vi "AlliGator Draw Phasor Ratio References on Phasor Plot.vi"(8 "error in (no error)":errorcluster, 9 "Overlay Group":string="Phasor Ratio References", 11 "Phasor Plot Refnum in":T1) -> (0 "error out":errorcluster, 3 "Phasor Plot Refnum out":T1)   [LabVIEW 2021, in "AlliGator Phasor Plot.lvlib"]
doc: "Does the actual drawing of Phasor Ratio References (and associated segment and boundary region) on the Phasor Plot image."
uses:
  AlliGator Phasor Plot.lvlib
  <vilib>/vision/Image Controls.llb/IMAQ Image.ctl
  Globals, Variables, Constants/AlliGator Variables List.ctl
  Phasor Ratio/AlliGator Phasor Plot Reference Points.ctl
  Settings/AlliGator Settings List.ctl
  08c29e31-a428-4f06-8fa9-37cc1cf687de.vi
  a2f43300-ec38-48b4-b16a-acb1cf69b6dd.vi
  Variant/Variant to Data/Variant to DBL.vi
  Variant/Variant to Data/Variant to I32.vi
  Variant/Variant to Data/Variant to Boolean.vi
  Globals, Variables, Constants/AlliGator Globals, Variables & Constants.lvlib
  Phasor Ratio/AlliGator Phasor Ratio.lvlib
  Settings/AlliGator Settings.lvlib
  Variant/Variant to Data/Variant to Data.lvlib
  Time/Time.lvlib
  Image/Image.lvlib
  Error/Error.lvlib
panel:
  out "elapsed (relative) seconds":dbl
  # "see the AlliGator License on the block diagram (Ctrl+E or Window:Show Block Diagram)"
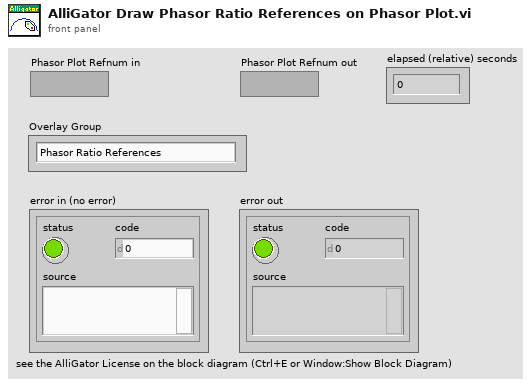
[diagram p1: front panel]
types:
  T1 = typedef "IMAQ Image.ctl" = refnum<image>
  T2 = typedef "IMAQ Point" = cluster{"X":sgl, "Y":sgl}
  T3 = typedef "AlliGator Settings.lvlib/AlliGator Settings List.ctl" = enum16{"GUI:Visible Settings Tab", "GUI:Last Run Version", "Source Image:Use Image Histogram for Contrast", "Source Image:Low Count Pixels Rejection Options", "Source Image:High Count Pixels Rejection Options", "Source Image:Use Image Brightness", "Source Image:Blend Overlay with Image Background", "Source Image:Use Fixed ROI Diameter", "Source Image:ROI Diameter", "Source Image:ROI Center Color", "Source Image:Peak Threshold", "Source Image:Intensity Threshold", "Source Image:Image Binning Options", "Source Image:Image Smoothing Options", "Source Image:Image Histogram Active", "Source Image:Invert Binary Mask", "Source Image:Hot Pixel Removal", "Source Image:Overlay Analyzed ROI Center", "Source Image:Auto-Adjust Contrast", "Source Image:Histogram Lower Percentile", "Source Image:Histogram Upper Percentile", "Source Image:Save Source Image", "Source Image:Scale Bar Options", "Source Image:Image Resolution (Pixel Size)", "Source Image:Flatfield Correction", "Source Image:Show Dead Left Columns Correction", "Source Image:Dead Left Columns Correction", "Source Image:Image Pre-Processing Operations Order", "Source Image:Overlay ROI Median", "Source Image:Median Overlay Color", "Data Information:Gate Width", "Data Information:Nanotime Gate Separation", "Data Information:Macrotime Gate Separation", "Data Information:Gate Step", "Data Information:# Gates", "Data Information:Gate Image Exposure", "Data Information:Gate Image Integration", "Data Information:Gates to Skip", "Data Information:Gates to Keep", "Data Information:Define Gates to", "Data Information:Channel Name", "Data Information:Available Channel Names", "Data Information:Channel Arithmetic", "Data Information:Background File Subtraction", "Data Information:Background File", "Data Information:Background Scaling Factor", "Data Information:Background Pile-up Correction", "Data Information:Background Pixel Well Capacity", "Data Information:Laser Period", "Data Information:SYNC Period", "Data Information:Pile-up Correction", "Data Information:Pixel Well Capacity", "Data Information:Dataset Scaling Factor", "Fluorescence Decay_Decay Pre-Processing:Reverse Gates", "Fluorescence Decay_Decay Pre-Processing:Verbose Decay Pre-Processing", "Fluorescence Decay_Decay Pre-Processing:Use Decay Pre-Processing", "Fluorescence Decay_Decay Pre-Processing:Background Subtraction", "Fluorescence Decay_Decay Pre-Processing:Background Definition Range", "Fluorescence Decay_Decay Pre-Processing:Baseline Subtraction Method", "Fluorescence Decay_Decay Pre-Processing:Decay Pre-Processing Operations Order", "Fluorescence Decay_Decay Pre-Processing:Smoothing Parameter", "Fluorescence Decay_Decay Pre-Processing:Shift Decay", "Fluorescence Decay_Decay Pre-Processing:Decay Shift Parameters", "Fluorescence Decay_Decay Pre-Processing:Fold Decay", "Fluorescence Decay_Decay Pre-Processing:# Folds", "Fluorescence Decay_Decay Pre-Processing:1-Normalize Decay", "Fluorescence Decay_Decay Pre-Processing:[0-1]-Normalize Decay", "Fluorescence Decay_Decay Pre-Processing:Smoothen Decay", "Fluorescence Decay_Decay Pre-Processing:Extrapolate Decay", "Fluorescence Decay_Decay Pre-Processing:Use Periodicity", "Fluorescence Decay_Decay Pre-Processing:Use Cursors", "Fluorescence Decay_Decay Pre-Processing:Tail Fraction", "Fluorescence Decay_Decay Pre-Processing:Head Fraction", "Fluorescence Decay_Decay Pre-Processing:Additional Points", "Fluorescence Decay_Decay Pre-Processing:Straighten Decay", "Fluorescence Decay_Decay Pre-Processing:Constant Background", "Fluorescence Decay_Decay Pre-Processing:Pixel-Normalize Decay", "Fluorescence Decay_Advanced Analysis:Extract IRF instead of Decay", "Fluorescence Decay_Advanced Analysis:IRF Extraction Options", "Fluorescence Decay_Advanced Analysis:IRF Optimization Options", "Fluorescence Decay_Advanced Analysis:Square Pulse Options", "Fluorescence Decay_Advanced Analysis:IRF Order", "Fluorescence Decay_Advanced Analysis:IRF Time Constants", "Fluorescence Decay_Advanced Analysis:Wavelet Analysis Options", "Fluorescence Decay_Advanced Analysis:Average Lifetime Options", "Fluorescence Decay_Fit Options:Fit Options", "Fluorescence Decay_Fit Options:Use Legacy Fitting Approach", "Fluorescence Decay_Fit Options:Use Data Information Laser Period", "Fluorescence Decay_Fit Parameters:Displayed Fit Parameters", "Fluorescence Decay_Fit Parameters:Fit Parameter Constraints", "Fluorescence Decay_Fit Parameters:Export Tabulated Results", "Fluorescence Decay_Fit Parameters:MLE Baseline Offset Type", "Fluorescence Decay_Fit Parameters:MLE Baseline Offset", "Fluorescence Decay_Fit Parameters:Guess Parameter Names", "Fluorescence Decay_Fit Parameters:Guess Parameter Values", "Fluorescence Decay_Fit Parameters:Guess Parameters Options", "Fluorescence Decay_Fit Parameters:Optimal Offset Selection Criterion", "Fluorescence Decay_Styles:Show Last Decay Only", "Fluorescence Decay_Styles:Decay Graph Color Array", "Fluorescence Decay:Decay Graph Active", "Fluorescence Decay Statistics:Min Peak Value", "Fluorescence Decay Statistics:Reject Low Decay Peak Pixels", "Fluorescence Decay Statistics:Reject High Decay Peak Pixels", "Fluorescence Decay Statistics:Max Peak Value", "Time Traces:Use File Timestamp", "Time Traces:Time Step", "Time Traces:Use Intensity Correction File", "Time Traces:Intensity Correction File", "Phasor Plot:Phasor Plot Smoothing Options", "Phasor Plot:Phasor Plot Size", "Phasor Plot:Phasor Plot Graphics Options", "Phasor Plot:Cumulative Phasor Plot", "Phasor Plot:Use Phasor Brightness", "Phasor Plot:Blend Overlay with Phasor Background", "Phasor Plot:Save Phasor Plot", "Phasor Plot:Show References", "Phasor Plot:Phasor Ratio Decay Range", "Phasor Plot:Exponential Fading", "Phasor Plot:Phasor Ratio Reference Colors", "Phasor Plot:Reference Radius", "Phasor Plot:Show Color Map Vertices", "Phasor Plot:Phasor Plot Active", "Phasor Plot:Phasor Ratio Color Map Type", "Phasor Plot:Phasor Ratio Color Map", "Phasor Plot:Phasor Ratio Display Range", "Phasor Plot:Selected Image ROI(s)", "Phasor Plot:All Image ROIs", "Phasor Plot:Selected Phasor Plot ROI(s)", "Phasor Plot:All Phasor Plot ROIs", "Phasor Plot:Phasor Ratio Color-Coded Quantity", "Phasor Plot:Store Phasor Harmonics", "Phasor Plot:Draw Reference Segment", "Phasor Plot:User-Defined Quantity", "Phasor Plot:Color Scale High Color", "Phasor Plot:Color Scale Low Color", "Phasor Plot:Intensity-weighted Phasor Plot", "Phasor Graph:Phasor Frequency", "Phasor Graph:Phasor Ratio Type", "Phasor Graph:Pixel-level Phasor Computation", "Phasor Graph:Save Phasor Graph", "Phasor Graph:Phasor Graph Active", "Phasor Graph:Phasor SDV Options", "Phasor Graph:Intensity-weighted Phasor Graph", "Phasor Graph:Define Shortest Lifetime as", "Phasor Calibration:Use Backup Calibration if needed", "Phasor Calibration:Backup Calibration Type", "Phasor Calibration:Calibration Type", "Phasor Calibration:Calibration Lifetime", "Phasor Calibration:Calibration Map Algorithm", "Single-Exponential Phasor Locus (SEPL):Gate Parameters", "Single-Exponential Phasor Locus (SEPL):User-defined Gate", "Single-Exponential Phasor Locus (SEPL):User-defined IRF", "Single-Exponential Phasor Locus (SEPL):Phasor Parameters", "Single-Exponential Phasor Locus (SEPL):Decay & IRF Parameters", "Single-Exponential Phasor Locus (SEPL):Display Parameters", "Lifetime Analysis:Decay Analysis Parameters", "Lifetime Analysis:Lifetime Map Active", "Plugins:Python Settings", "Miscellaneous:Verbose Mode", "Miscellaneous:Beep after Script", "Miscellaneous:Saved Image File Format", "Miscellaneous:Exported Gate Image Settings", "Miscellaneous:Include Loading in Timing", "Miscellaneous:Verbose Settings Mode", "Miscellaneous:Histogram Options", "Miscellaneous:Beep on Error", "Miscellaneous:# Logical Processors Used", "Miscellaneous:ROI Description Max Characters", "Miscellaneous:Verbose Error Mode", "Miscellaneous:Transparent Mask Color"}
  T4 = cluster{"Reference 1":u32, "Reference 2":u32, "Boundary":u32}
  T5 = typedef "AlliGator Phasor Ratio.lvlib/AlliGator Phasor Plot Reference Points.ctl" = cluster{"O_h":dbl, "O_v":dbl, "1_h":dbl, "1_v":dbl}
  T6 = typedef "AlliGator Globals, Variables & Constants.lvlib/AlliGator Variables List.ctl" = enum16{"---- GUI ----", "GUI:Initialization Status", "GUI:State Indicators Refnum", "GUI:Original AlliGator Menu Items", "GUI:Current Action Loop State", "GUI:Script in progress", "GUI:Playback", "GUI:Loop Playback", "GUI:Search ROI Used", "GUI:Search ROI", "Decay Graph Max Legend Size", "Intensity Graph Max Legend Size", "Decay Statistics Graph Max Legend Size", "Phasor Graph Max Legend Size", "Phasor Ratio Graph Max Legend Size", "Lifetime Graph Max Legend Size", "---- Files ----", "Files:Export Dataset Frames as Individual Files", "Files:Show Batch Export Help Balloons", "Files:Frames in Dataset", "Files:ptu File Frame Start Indices", "Files:Current Frame in Dataset", "Files:Current Frame Timestamp", "Files:Dataset Loaded", "Files:Dataset Metadata", "Files:Dataset Channel", "Files:Dataset Data Description", "Files:Background Dataset Metadata", "Files:Background Dataset Channel", "Files:Background Dataset Data Description", "Files:Background File Subtraction", "Files:Background File Path", "Files:Background File Pile-up Correction", "Files:Background File Pixel Well Capacity", "Files:Background File Scaling Factor", "Files:Current Dataset Load Settings", "Files:Dataset Path", "Files:ICCD-specific Information", "Files:Macrotime Gate Separation", "------ Python Plugins ------", "Python Plugins:Information", "Python Plugins:Python Session", "Python Plugins:Valid Python Session?", "---- Source Image ----", "Source Image:ROIs", "Source Image:Current ROI", "Source Image:ROI Event Refnum", "X_Source Image:Display Range", "X_Source Image:Palette Information", "X_Source Image:Type of Displayed Image", "X_Time Gate Slider", "Source Image:Palette List", "Source Image:Scale", "Source Image:ROI Overlay Color", "Source Image:Overlay to Erase", "Source Image:Is Displayed Image Accumulated", "Source Image:White Light Image Modified", "Source Image:Mask Image Modified", "---- Image Profile Window ----", "Image Profile:Window Event Refnum", "Image Profile:IntensityType", "Image Profile:Intensity Average Type", "Image Profile:Intensity-weighted SDV", "Image Profile:Box Profile Type", "Image Profile:Window Open", "Image Profile:Plotted Fit Parameter", "------ Phasor Graph -------", "Phasor Graph:Show Line", "---- Phasor Plot ---", "Phasor Plot:Parameters Changed", "Phasor Plot:FLI Dataset Modified since last Calculation", "Phasor Harmonics Data", "Selected Phasor Harmonics", "Phasor Harmonic Manager Event Refnum", "Phasor Plot:ROIs", "Phasor Plot:Current ROI", "Phasor Plot:ROI Event Refnum", "Phasor Plot:Image Reference Points", "Phasor Plot:Computed", "Phasor Plot:Palette Information", "Phasor Plot:Palette List", "Phasor Plot:Phasor Ratio Palette Information", "Phasor Plot:Phasor Ratio Palette List", "Phasor Plot:Image Scale", "Phasor Plot:Image Overlay to Erase", "Phasor Plot:Image Elements to Update", "Phasor Plot:Current Calculation Parameters", "Phasor Plot:Current Calibration Options", "Phasor Plot:Reset Cumulated Phasor Plot", "Phasor Plot:Reference 1", "Phasor Plot:Lifetime Reference 1", "Phasor Plot:Reference 1 Frequency", "Phasor Plot:Reference 2", "Phasor Plot:Lifetime Reference 2", "Phasor Plot:Reference 2 Frequency", "---- Decay Analysis ----", "Number of Selected Decays to Fit", "LS Fit Results", "LAR Fit Results", "BS Fit Results", "Last Decay Max - Min", "Best Fit Parameters", "Best Fit Parameter Names", "Actual Size X", "Actual Size Y", "Binning X", "Binning Y", "Actual # Gates", "Dataset Number", "Gates to...", "Gates Skipped", "Gates to keep", "Gate Step", "Gate Separation", "Reversed Gates", "Pile-up Correction", "Pixel Well Capacity", "Background Subtracted", "Background Subtraction Method", "Background Definition Range", "Background File (deprecated)", "Number of Dataset Accumulated", "Array of Accumulated Dataset Paths", "Do Averaged Datasets", "Destination File Path", "Process Plot Target", "Use 1/D as Phasor Frequency", "---- Decay Fit Parameter Map -----", "Decay Fit Parameter Map:Palette Information", "Decay Fit Parameter Map:Palette List", "Decay Fit Parameter Map:X Resolution", "Decay Fit Parameter Map:Y Resolution", "Decay Fit Parameter Map:Use Decay Fit Result Constraints", "Decay Fit Parameter Map:Decay Fit Result Constraints", "Decay Fit Parameter Map:Decay Fit Result Constraints Applied", "---- Parameter Map ----", "Parameter Map:Palette Information", "Parameter Map:Palette List", "------- Local Decay Window ---------", "Local Decay Graph Window:Event Refnum", "Local Decay Graph Window:Use normalized IRF for convolution", "----- Miscellaneous ----", "Misc:Skippable Dialog Windows Status"}
  T7 = typedef "Phasor.lvlib/Phasor (g, s).ctl" = cluster{"g":dbl, "s":dbl}
  T8 = cluster{"Phasor Plot x":dbl, "Phasor Plot y":dbl}
  T9 = cluster{"Left":i32, "Top":i32, "Right":i32, "Bottom":i32}
  T10 = cluster{"Phasor Plot x":dbl, "Phasor Plot y":dbl}[]
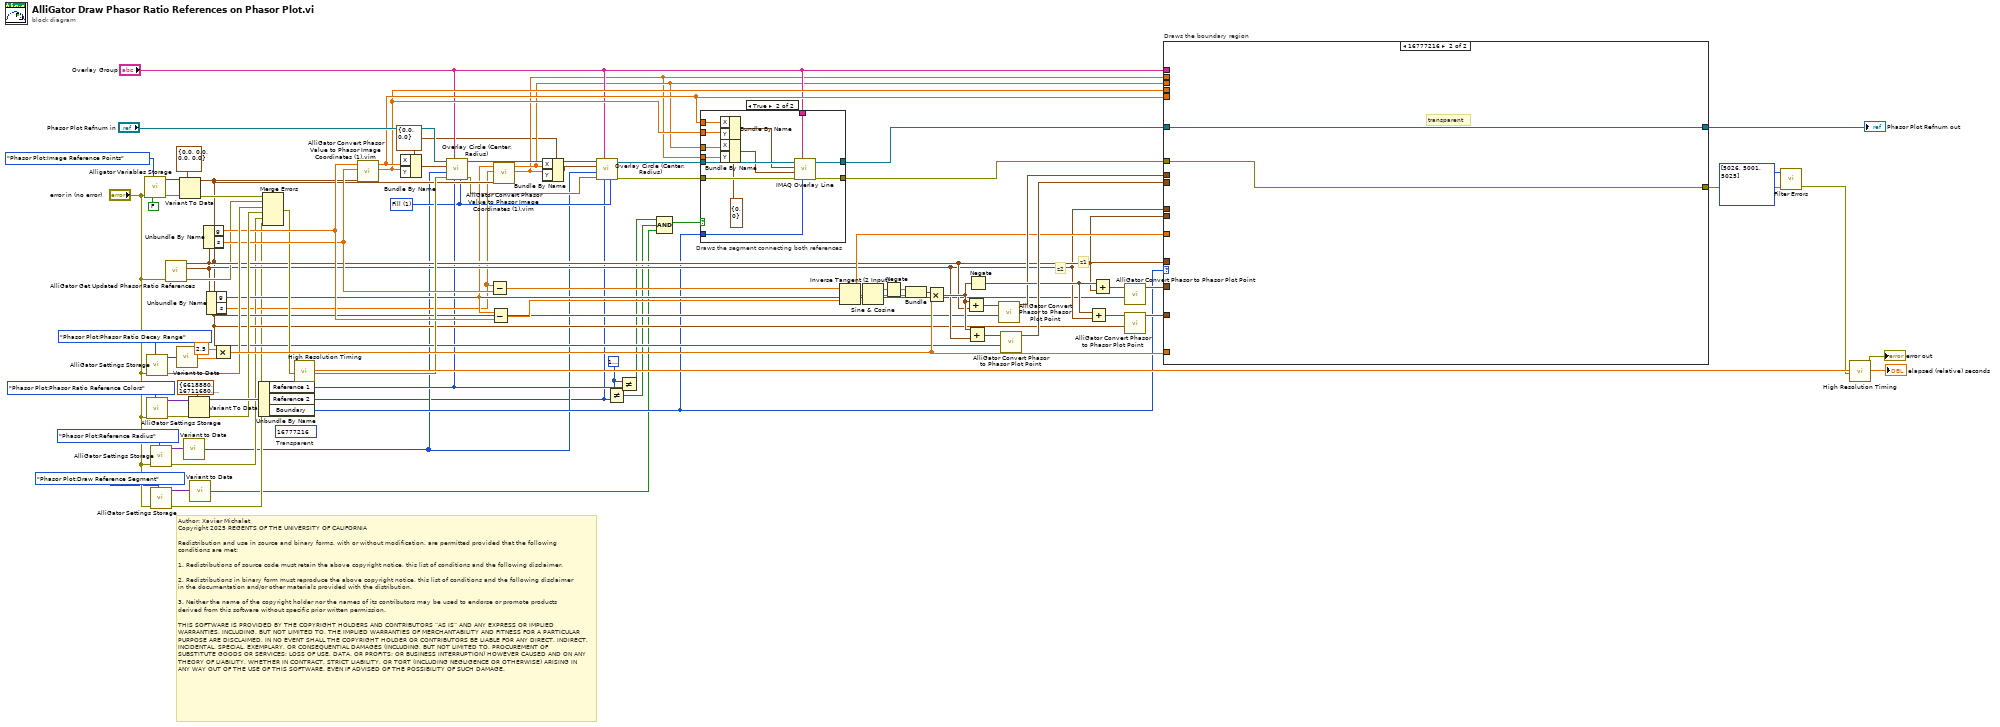
[diagram p0: block diagram]
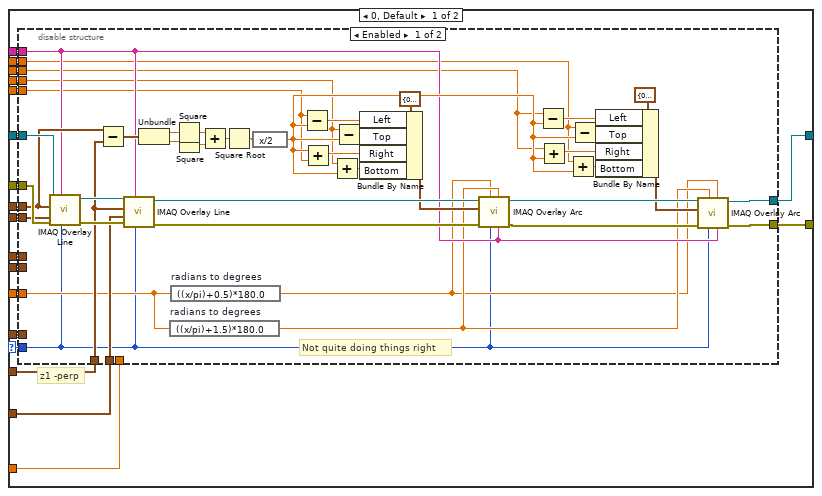
[diagram p3: hidden frame]
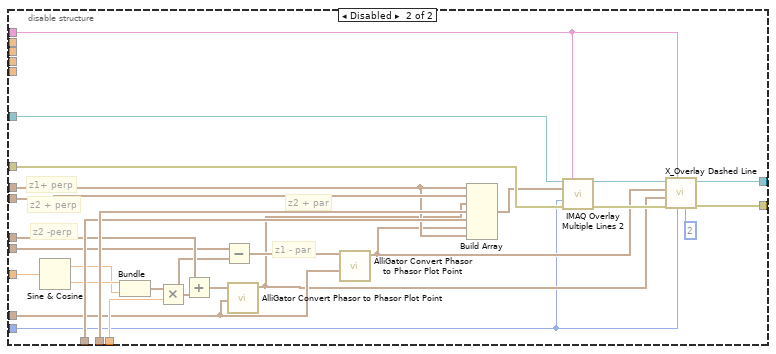
[diagram p4: hidden frame]
diagram:
  w3 = u32 1 items=["Frame", "Fill"] ("Drawing Mode (Frame)")
  w15 = u32 16777216 ("Color")
  w5 = T2 {"X"=0.0, "Y"=0.0} ("Center")
  (unwired) u32 16777216  # Transparent
  # "Author: Xavier Michalet\nCopyright 2025 REGENTS OF THE UNIVERSITY OF CALIFORNIA\n\nRedistribution and use in source and binary forms, with or without modification, are permitted provided that the following conditions are met:\n\n1. Redistributions of source code must retain the above copyright notice, this list of conditions and the following disclaimer.\n\n2. Redistributions in binary form must reproduce the above copyright notice, this list of conditions and the following disclaimer in the documentation and/or other materials provided with the distribution.\n\n3. Neither the name of the copyright holder nor the names of its contributors may be used to endorse or promote products derived from this software without specific prior written permission.\n\nTHIS SOFTWARE IS PROVIDED BY THE COPYRIGHT HOLDERS AND CONTRIBUTORS “AS IS” AND ANY EXPRESS OR IMPLIED WARRANTIES, INCLUDING, BUT NOT LIMITED TO, THE IMPLIED WARRANTIES OF MERCHANTABILITY AND FITNESS FOR A PARTICULAR PURPOSE ARE DISCLAIMED. IN NO EVENT SHALL THE COPYRIGHT HOLDER OR CONTRIBUTORS BE LIABLE FOR ANY DIRECT, INDIRECT, INCIDENTAL, SPECIAL, EXEMPLARY, OR CONSEQUENTIAL DAMAGES (INCLUDING, BUT NOT LIMITED TO, PROCUREMENT OF SUBSTITUTE GOODS OR SERVICES; LOSS OF USE, DATA, OR PROFITS; OR BUSINESS INTERRUPTION) HOWEVER CAUSED AND ON ANY THEORY OF LIABILITY, WHETHER IN CONTRACT, STRICT LIABILITY, OR TORT (INCLUDING NEGLIGENCE OR OTHERWISE) ARISING IN ANY WAY OUT OF THE USE OF THIS SOFTWARE, EVEN IF ADVISED OF THE POSSIBILITY OF SUCH DAMAGE."
  # "z2"
  # "z1"
  n1 = call "Alligator Variables Storage.vi"("Get(F)/Set"=FALSE, "AlliGator Variable"=AlliGator_Variables_List."Phasor Plot:Image Reference Points" ("Alligator Variable"), "Error In"="error in (no error)") -> ("Error Out"=w82:errorcluster, "Data out"=w83:variant)  [unwired: 6 in, 1 out]
  n2 = call "AlliGator Settings Storage.vi"("AlliGator Settings List"=AlliGator_Settings_List."Phasor Plot:Phasor Ratio Decay Range", "Error In"="error in (no error)") -> ("Error Out"=w64:errorcluster, "Variant Data out"=w78:variant)  [unwired: 8 in]
  n3 = call "AlliGator Settings Storage.vi"("AlliGator Settings List"=AlliGator_Settings_List."Phasor Plot:Phasor Ratio Reference Colors", "Error In"="error in (no error)") -> ("Error Out"=w70:errorcluster, "Variant Data out"=w72:variant)  [unwired: 8 in]
  n4 = call "AlliGator Settings Storage.vi"("AlliGator Settings List"=AlliGator_Settings_List."Phasor Plot:Draw Reference Segment", "Error In"="error in (no error)") -> ("Error Out"=w25:errorcluster, "Variant Data out"=w27:variant)  [unwired: 8 in]
  n5 = call "AlliGator Settings Storage.vi"("AlliGator Settings List"=AlliGator_Settings_List."Phasor Plot:Reference Radius", "Error In"="error in (no error)") -> ("Error Out"=w34:errorcluster, "Variant Data out"=w35:variant)  [unwired: 8 in]
  n6 = call "AlliGator Get Updated Phasor Ratio References.vi"("error in (no error)"="error in (no error)") -> ("error out"=w39:errorcluster, "Phasor Ratio Reference 2"=w38:T7, "Phasor Ratio Reference 1"=w40:T7)  [unwired: 8 in]
  n7 = call-poly "Variant to Data.vi"("Variant"=w78) -> ("Value"=w75:dbl)  [unwired: 8 in]
  n8 = Variant To Data(error in=w82, type=T5 {"O_h"=0.0, "O_v"=0.0, "1_h"=0.0, "1_v"=0.0} ("Phasor Plot Reference Points"), Variant=w83) -> (data=w37:T5, error out=w65:errorcluster)
  n9 = call-poly "Variant to Data.vi"("Variant"=w35) -> ("Value"=w2:i32)  [unwired: 8 in]
  n10 = Variant To Data(error in=w70, type=T4 {"Reference 1"=6618880, "Reference 2"=16711680, "Boundary"=16776960} ("Phasor Ratio Reference Colors"), Variant=w72) -> (data=w69:T4, error out=w63:errorcluster)
  n11 = call-poly "Variant to Data.vi"("Variant"=w27) -> ("Value"=w16:bool)  [unwired: 8 in]
  n12 = Unbundle By Name(w40) -> ("g"=w62:dbl, "s"=w61:dbl)
  n13 = Unbundle By Name(w38) -> ("g"=w30:dbl, "s"=w29:dbl)
  n14 = Multiply(x=2.5, y=w75) -> (x*y=w74:dbl)
  n15 = Unbundle By Name(w69) -> ("Reference 1"=w17:u32, "Reference 2"=w1:u32, "Boundary"=w23:u32)
  n16 = Merge Errors(w65, w39, w64, w63, w34, w25) -> (w43:errorcluster)
  n17 = call "High Resolution Timing.vi"("Error In"=w43) -> ("elapsed (relative) seconds"=w68:dbl, "Error Out"=w42:errorcluster)  [unwired: 16 in, 1 out]
  n18 = call "AlliGator Convert Phasor Value to Phasor Image Coordinates (1).vim"("Phasor Plot Reference Points"=w37, "Phasor s"=w61, "Phasor g"=w62) -> ("Phasor Plot y"=w19:dbl, "Phasor Plot x"=w20:dbl)  [unwired: 7 in]
  n19 = Bundle By Name(cluster=w5, "X"=w20, "Y"=w19) -> (w18:T2)
  n20 = call "Overlay Circle (Center, Radius).vi"("Drawing Mode (Frame)"=w3, "Color"=w17, "Overlay Group"="Overlay Group", "error in (no error)"=w42, "Radius"=w2, "Center"=w18, "Image Refnum in"="Phasor Plot Refnum in") -> ("error out"=w10:errorcluster, "Image Refnum out"=w12:T1)  [unwired: 3 in]
  n21 = Subtract(x=w29, y=w61) -> (x-y=w60:dbl)
  n22 = Subtract(x=w30, y=w62) -> (x-y=w59:dbl)
  n23 = call "AlliGator Convert Phasor Value to Phasor Image Coordinates (1).vim"("Phasor Plot Reference Points"=w37, "Phasor s"=w29, "Phasor g"=w30) -> ("Phasor Plot y"=w6:dbl, "Phasor Plot x"=w7:dbl)  [unwired: 7 in]
  n24 = Bundle By Name(cluster=w5, "X"=w7, "Y"=w6) -> (w4:T2)
  n25 = call "Overlay Circle (Center, Radius).vi"("Drawing Mode (Frame)"=w3, "Color"=w1, "Overlay Group"="Overlay Group", "error in (no error)"=w10, "Radius"=w2, "Center"=w4, "Image Refnum in"=w12) -> ("error out"=w9:errorcluster, "Image Refnum out"=w11:T1)  [unwired: 3 in]
  n26 = Not Equal?(x=w15, y=w1) -> (x != y?=w14:bool)
  n27 = Not Equal?(x=w15, y=w17) -> (x != y?=w13:bool)
  n28 = Compound Arithmetic op=AND(w13, w14, w16) -> (w24:bool)
  n29 = case "Draws the segment connecting both references" shown="True" w24 {
    tunnel: w23 -> [_ w95]
    tunnel: w19 -> [_ w93]
    tunnel: w11 -> [w86 w99]
    tunnel: [w86 w98] -> w22
    tunnel: w9 -> [w85 w97]
    tunnel: [w85 w96] -> w21
    tunnel: w20 -> [_ w94]
    tunnel: w7 -> [_ w92]
    tunnel: w6 -> [_ w91]
    tunnel: "Overlay Group" -> [_ w87]
    frame False {
    }
    frame True {
      w90 = cluster{"X":i32, "Y":i32} {"X"=0, "Y"=0} ("Start Point")
      n30 = Bundle By Name(cluster=w90, "X"=w94, "Y"=w93) -> (w89:cluster{"X":i32, "Y":i32})
      n31 = Bundle By Name(cluster=w90, "X"=w92, "Y"=w91) -> (w88:cluster{"X":i32, "Y":i32})
      n32 = call "IMAQ Overlay Line"("Color"=w95, "Group"=w87, "error in (no error)"=w97, "End Point"=w88, "Start Point"=w89, "Image"=w99) -> ("error out"=w96:errorcluster, "Image Out"=w98:T1)  [unwired: 4 in]
    }
  }
  n33 = Inverse Tangent (2 Input)(1:w59, 2:w60) -> (0:w44:dbl)
  n34 = Sine & Cosine(0:w44) -> (1:w58:dbl, 2:w57:dbl)
  n35 = Negate(x=w58) -> (-x=w56:dbl)
  n36 = Bundle(w56, w57) -> (w55:cluster{dbl, dbl})  [unwired: 1 in]
  n37 = Multiply(x=w55, y=w74) -> (x*y=w54:cluster{dbl, dbl})
  n38 = Add(x=w54, y=w40) -> (x+y=w53:T7)
  n39 = Add(x=w54, y=w38) -> (x+y=w52:T7)
  n40 = Negate(x=w54) -> (-x=w49:cluster{dbl, dbl})
  n41 = call "AlliGator Convert Phasor to Phasor Plot Point.vi"("Phasor Plot Reference Points"=w37, "Phasor"=w53) -> ("Phasor Plot Point"=w46:T8)  [unwired: 9 in]
  n42 = call "AlliGator Convert Phasor to Phasor Plot Point.vi"("Phasor Plot Reference Points"=w37, "Phasor"=w52) -> ("Phasor Plot Point"=w51:T8)  [unwired: 9 in]
  n43 = Add(x=w49, y=w38) -> (x+y=w48:T7)
  n44 = Add(x=w49, y=w40) -> (x+y=w50:T7)
  n45 = call "AlliGator Convert Phasor to Phasor Plot Point.vi"("Phasor Plot Reference Points"=w37, "Phasor"=w50) -> ("Phasor Plot Point"=w45:T8)  [unwired: 9 in]
  n46 = call "AlliGator Convert Phasor to Phasor Plot Point.vi"("Phasor Plot Reference Points"=w37, "Phasor"=w48) -> ("Phasor Plot Point"=w47:T8)  [unwired: 9 in]
  n47 = case "Draws the boundary region" shown="16777216" w23 {
    selector: w23 -> [w116 _]
    tunnel: [w118 w190] -> w76
    tunnel: w74 -> [w117 _]
    tunnel: "Overlay Group" -> [w115 _]
    tunnel: w22 -> [w114 w190]
    tunnel: w21 -> [w113 w189]
    tunnel: w51 -> [w112 _]
    tunnel: w47 -> [w111 _]
    tunnel: w46 -> [w110 _]
    tunnel: w45 -> [w109 _]
    tunnel: w44 -> [w108 _]
    tunnel: [w107 w189] -> w32
    tunnel: w40 -> [w106 _]
    tunnel: w38 -> [w105 _]
    tunnel: w37 -> [w104 _]
    tunnel: w20 -> [w103 _]
    tunnel: w19 -> [w102 _]
    tunnel: w7 -> [w101 _]
    tunnel: w6 -> [w100 _]
    frame 0, Default {
      # "z1 -perp"
      n48 = disable-structure shown="Enabled" {
        disable-tunnel: w114 -> [w161 w173]
        disable-tunnel: w113 -> [w160 w172]
        disable-tunnel: w112 -> [w157 w188]
        disable-tunnel: w111 -> [w156 w187]
        disable-tunnel: w110 -> [w151 w185]
        disable-tunnel: w109 -> [w150 w186]
        disable-tunnel: w103 -> [w119 _]
        disable-tunnel: w102 -> [w120 _]
        disable-tunnel: w108 -> [w138 w184]
        disable-tunnel: w101 -> [w121 _]
        disable-tunnel: w100 -> [w122 _]
        disable-tunnel: w115 -> [w128 w169]
        disable-tunnel: [w127 w167] -> w107
        disable-tunnel: [w126 w166] -> w118
        disable-tunnel: w116 -> [w123 w163]
        disable-tunnel: w106 -> [_ w177]
        disable-tunnel: w117 -> [_ w180]
        disable-tunnel: w105 -> [_ w179]
        disable-tunnel: w104 -> [_ w174]
        frame Enabled {
          # "Not quite doing things right"
          n49 = call "IMAQ Overlay Line"("Color"=w123, "Group"=w128, "error in (no error)"=w160, "End Point"=w157, "Start Point"=w151, "Image"=w161) -> ("error out"=w158:errorcluster, "Image Out"=w159:T1)  [unwired: 4 in]
          n50 = Subtract(x=w151, y=w150) -> (x-y=w149:T8)
          n51 = call "IMAQ Overlay Line"("Color"=w123, "Group"=w128, "error in (no error)"=w158, "End Point"=w156, "Start Point"=w150, "Image"=w159) -> ("error out"=w154:errorcluster, "Image Out"=w155:T1)  [unwired: 4 in]
          n52 = Unbundle(w149) -> ("Phasor Plot x"=w148:dbl, "Phasor Plot y"=w147:dbl)
          n53 = expression code="((x/pi)+1.5)*180.0" "radians to degrees"(w138) -> (w125:dbl)
          n54 = expression code="((x/pi)+0.5)*180.0" "radians to degrees"(w138) -> (w124:dbl)
          n55 = Square(x=w148) -> (x^2=w146:dbl)
          n56 = Square(x=w147) -> (x^2=w145:dbl)
          n57 = Add(x=w146, y=w145) -> (x+y=w144:dbl)
          n58 = Square Root(x=w144) -> (sqrt(x)=w140:dbl)
          n59 = expression code="x/2"(w140) -> (w133:dbl)
          n60 = Subtract(x=w119, y=w133) -> (x-y=w143:dbl)
          n61 = Add(x=w133, y=w119) -> (x+y=w142:dbl)
          n62 = Add(x=w120, y=w133) -> (x+y=w139:dbl)
          n63 = Subtract(x=w120, y=w133) -> (x-y=w141:dbl)
          n64 = Bundle By Name(cluster=T9 {"Left"=0, "Top"=0, "Right"=0, "Bottom"=0} ("Bounding Rectangle"), "Left"=w143, "Top"=w141, "Right"=w142, "Bottom"=w139) -> (w152:T9)
          n65 = call "IMAQ Overlay Arc"("Group"=w128, "End Angle (degrees)"=w125, "Color"=w123, "Start Angle (degrees)"=w124, "error in (no error)"=w154, "Bounding Rectangle"=w152, "Image"=w155) -> ("error out"=w129:errorcluster, "Image Out"=w131:T1)  [unwired: 3 in]
          n66 = Subtract(x=w121, y=w133) -> (x-y=w134:dbl)
          n67 = Add(x=w121, y=w133) -> (x+y=w135:dbl)
          n68 = Add(x=w122, y=w133) -> (x+y=w137:dbl)
          n69 = Subtract(x=w122, y=w133) -> (x-y=w136:dbl)
          n70 = Bundle By Name(cluster=T9 {"Left"=0, "Top"=0, "Right"=0, "Bottom"=0} ("Bounding Rectangle"), "Left"=w134, "Top"=w136, "Right"=w135, "Bottom"=w137) -> (w130:T9)
          n71 = call "IMAQ Overlay Arc"("Group"=w128, "End Angle (degrees)"=w124, "Color"=w123, "Start Angle (degrees)"=w125, "error in (no error)"=w129, "Bounding Rectangle"=w130, "Image"=w131) -> ("error out"=w127:errorcluster, "Image Out"=w126:T1)  [unwired: 3 in]
        }
        frame Disabled {
          # "z2 + par"
          # "z1 - par"
          # "z1+ perp"
          # "z2 + perp"
          # "z2 -perp"
          n72 = Sine & Cosine(0:w184) -> (1:w182:dbl, 2:w183:dbl)
          n73 = Bundle(w183, w182) -> (w181:cluster{dbl, dbl})  [unwired: 1 in]
          n74 = Multiply(x=w181, y=w180) -> (x*y=w176:cluster{dbl, dbl})
          n75 = Add(x=w179, y=w176) -> (x+y=w178:T7)
          n76 = Subtract(x=w177, y=w176) -> (x-y=w175:T7)
          n77 = call "AlliGator Convert Phasor to Phasor Plot Point.vi"("Phasor Plot Reference Points"=w174, "Phasor"=w178) -> ("Phasor Plot Point"=w164:T8)  [unwired: 9 in]
          n78 = call "AlliGator Convert Phasor to Phasor Plot Point.vi"("Phasor Plot Reference Points"=w174, "Phasor"=w175) -> ("Phasor Plot Point"=w165:T8)  [unwired: 9 in]
          n79 = Build Array(w185, w188, w164, w187, w186, w165, w185) -> (w171:T10)
          n80 = call "IMAQ Overlay Multiple Lines 2"("Image"=w173, "Group"=w169, "Line End Points"=w171, "Color"=w163, "error in (no error)"=w172) -> ("Image Out"=w170:T1, "error out"=w168:errorcluster)  [unwired: 9 in]
          n81 = call "X_Overlay Dashed Line.vi"("Dash Length (0)"=u32 2, "Color"=w163, "Overlay Group"=w169, "error in (no error)"=w168, "Point 2"=w164, "Point 1"=w165, "Refnum in"=w170) -> ("error out"=w167:errorcluster, "Refnum out"=w166:T1)  [unwired: 3 in]
        }
      }
    }
    frame 16777216 {
      # "transparent"
    }
  }
  "Phasor Plot Refnum out" <- w76
  n82 = call "Filter Errors.vi"("Filtered Errors"=i32[] [5026, 5001, 5025], "error in (no error)"=w32) -> ("error out"=w31:errorcluster)  [unwired: 7 in]
  n83 = call "High Resolution Timing.vi"("relative seconds (NaN)"=w68, "Error In"=w31) -> ("elapsed (relative) seconds"=→"elapsed (relative) seconds":dbl, "Error Out"=→"error out":errorcluster)  [unwired: 15 in, 1 out]
